vi "Relink_Mutation.vi"(0 "Diagram":refnum<vi>, 5 "ObjRef":refnum<vi>, 6 "Kind":string="SubVI", 7 "Information":string="<Not A Path>") -> (3 "Replace?":bool)   [LabVIEW 2020]
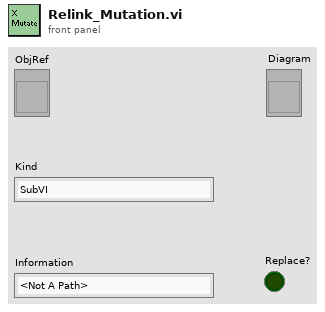
[diagram p1: front panel]
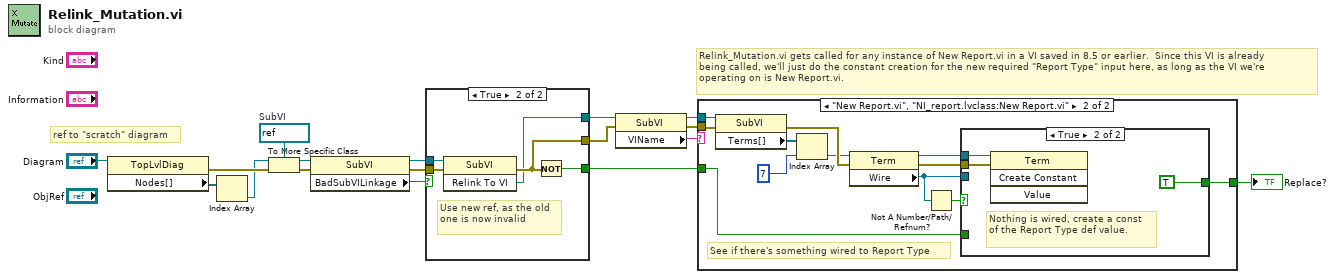
[diagram p0: block diagram]
diagram:
  w11 = refnum<vi> refnum  # SubVI
  # "Relink_Mutation.vi gets called for any instance of New Report.vi in a VI saved in 8.5 or earlier.  Since this VI is already\nbeing called, we'll just do the constant creation for the new required \"Report Type\" input here, as long as the VI we're \noperating on is New Report.vi."
  # "ref to \"scratch\" diagram"
  n1 = property class="TopLvlDiag"(reference="Diagram") -> (error out=w17:errorcluster, "Nodes[]"=w10:refnum<vi>[])  [unwired: 1 in, 1 out]
  n2 = Index Array(array=w10) -> (element=w9:refnum<vi>)  [unwired: 1 in]
  n3 = To More Specific Class(target class=w11, reference=w9, error in=w17) -> (specific class reference=w8:refnum<vi>, error out=w16:errorcluster)
  n4 = property class="SubVI"(reference=w8, error in=w16) -> (reference out=w7:refnum<vi>, error out=w15:errorcluster, "BadSubVILinkage"=w6:bool)
  n5 = case shown="True" w6 {
    tunnel: w7 -> [w18 w22]
    tunnel: w15 -> [w19 w24]
    tunnel: [_ w21] -> w3
    tunnel: [w19 w23] -> w13
    tunnel: [w18 w20] -> w2
    frame False {
      # "don't relink if linkage is good"
    }
    frame True {
      # "Use new ref, as the old one is now invalid"
      n6 = invoke class="SubVI" method="Relink To VI"(reference=w22, error in=w24) -> (error out=w23:errorcluster, "Relink To VI"=w20:refnum<vi>)  [unwired: 1 in, 1 out]
      n7 = Not(x=w23) -> (.not. x?=w21:bool)
    }
  }
  n8 = property class="SubVI"(reference=w2, error in=w13) -> (reference out=w4:refnum<vi>, error out=w14:errorcluster, "VIName"=w5:string)
  n9 = case shown="\"New Report.vi\", \"NI_report.lvclass:New Report.vi\"" w5 {
    tunnel: w14 -> [_ w37]
    tunnel: w4 -> [_ w34]
    tunnel: [w25 w27] -> w1
    tunnel: w3 -> [w25 w28]
    frame Default {
      # "This is not New Report.vi.  We're done mutating."
    }
    frame "New Report.vi", "NI_report.lvclass:New Report.vi" {
      # "See if there's something wired to Report Type"
      n10 = property class="SubVI"(reference=w34, error in=w37) -> (error out=w36:errorcluster, "Terms[]"=w33:refnum<vi>[])  [unwired: 1 out]
      n11 = Index Array(array=w33, index=7) -> (element=w32:refnum<vi>)
      n12 = property class="Term"(reference=w32, error in=w36) -> (reference out=w29:refnum<vi>, error out=w35:errorcluster, "Wire"=w30:refnum<vi>)
      n13 = Not A Number/Path/Refnum?(number/path/refnum=w30) -> (NaN/Path/Refnum?=w31:bool)
      n14 = case shown="True" w31 {
        tunnel: w30 -> [_ _]
        tunnel: w29 -> [_ w40]
        tunnel: w35 -> [_ w41]
        tunnel: w28 -> [w38 _]
        tunnel: [w38 TRUE] -> w27
        frame False {
          # "Something is wired...do nothing."
        }
        frame True {
          # "Nothing is wired, create a const\nof the Report Type def value."
          n15 = invoke class="Term" method="Create Constant"(reference=w40, error in=w41) -> ()  [unwired: 2 in, 4 out]
        }
      }
    }
  }
  "Replace?" <- w1
